vi "---Config Interface.vi"(7 "Config Data":T1 {"Step Duration" max=99999 step=1}, 8 "error in (no error)":errorcluster, 9 "Stop":bool, 10 "Config Command":T2, 11 "Config Model":T3) -> (0 "error out":errorcluster)   [LabVIEW 2017]
uses:
  Controls/Congif Data.ctl
  Controls/Config Commands.ctl
  Controls/Config Model.ctl
panel:
  out "Configuration Data records":string
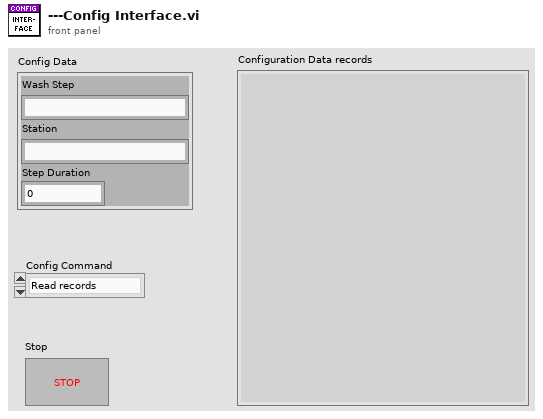
[diagram p1: front panel]
types:
  T1 = typedef "Congif Data.ctl" = cluster{"Wash Step":string, "Station":string, "Step Duration":u32}
  T2 = typedef "Config Commands.ctl" = enum16{"Read records", "Query timing data", "Insert new data records", "Update data records"}
  T3 = typedef "Config Model.ctl" = cluster{"Config Event":refnum<user-event>, "Config DVR":refnum<data-value>, "Config CMD":refnum<user-event>, "Config Locked?":refnum<data-value>}
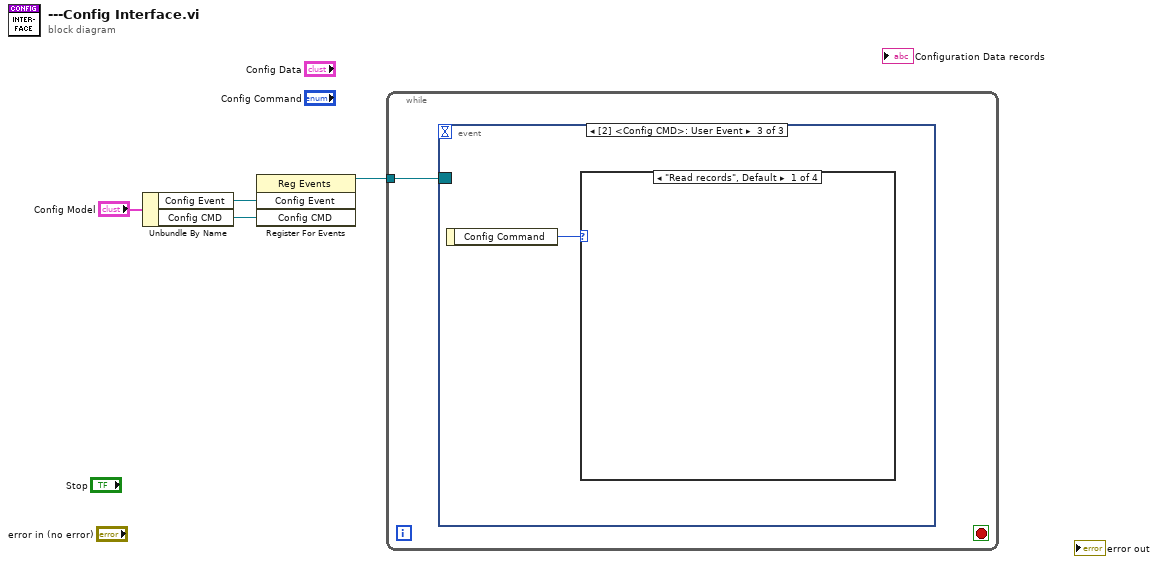
[diagram p0: block diagram]
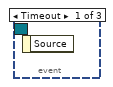
[diagram p2: hidden frame]
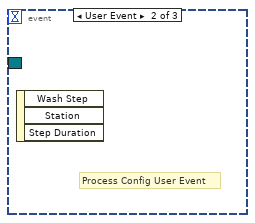
[diagram p3: hidden frame]
diagram:
  n1 = Unbundle By Name("Config Model") -> ("Config Event"=w3:refnum<user-event>, "Config CMD"=w2:refnum<user-event>)
  n2 = register-events(w3, w2) -> (reference out=w1:refnum<event-registration>)  [unwired: 2 in, 1 out]
  n3 = while {
    tunnel: w1 -> [w5]
    stop <- _ stop-if-true
    n4 = event shown="[2] <Config CMD>: User Event" {
      selector: w5 -> [_ _ _]
      dyn-events: _ -> [_ _ _]
      timeout: _ -> [_ _ _]
      event Timeout {
        n5 = event-data() -> ()  [unwired: 1 in, 1 out]
      }
      event User Event {
        # "Process Config User Event"
        n6 = event-data() -> ()  [unwired: 1 in, 3 out]
      }
      event User Event {
        n7 = event-data() -> ("Config Command"=w6:T2)  [unwired: 1 in]
        n8 = case shown="\"Read records\", Default" w6 {
          frame "Read records", Default {
          }
          frame "Query timing data" {
          }
          frame "Insert new data records" {
          }
          frame "Update data records" {
          }
        }
      }
    }
  }
